vi "Emballage_BDD_lecture_Table_Correspondance_GVF_Index.vi"(10 "Column Names en entrée":string[](array[string]), 11 "Énum":enum16{"get", "set"}(ring)) -> (3 "Cluster_index_champs_correspondance":T1)   [LabVIEW 2020]
uses:
  Emballage_Index_correspondance.ctl
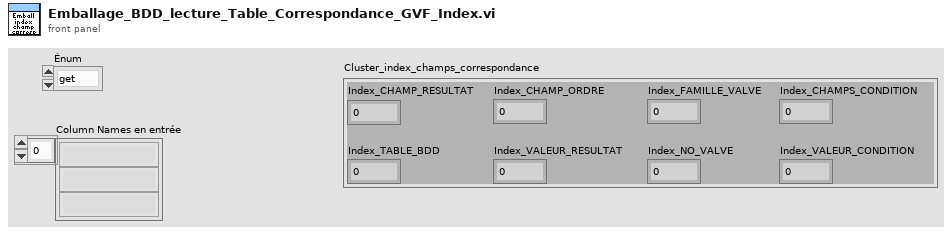
[diagram p1: front panel]
types:
  T1 = typedef "Emballage_Index_correspondance.ctl" = cluster{"Index_CHAMP_RESULTAT":i32, "Index_TABLE_BDD":i32, "Index_CHAMP_ORDRE":i32, "Index_VALEUR_RESULTAT":i32, "Index_FAMILLE_VALVE":i32, "Index_NO_VALVE":i32, "Index_CHAMPS_CONDITION":i32, "Index_VALEUR_CONDITION":i32}
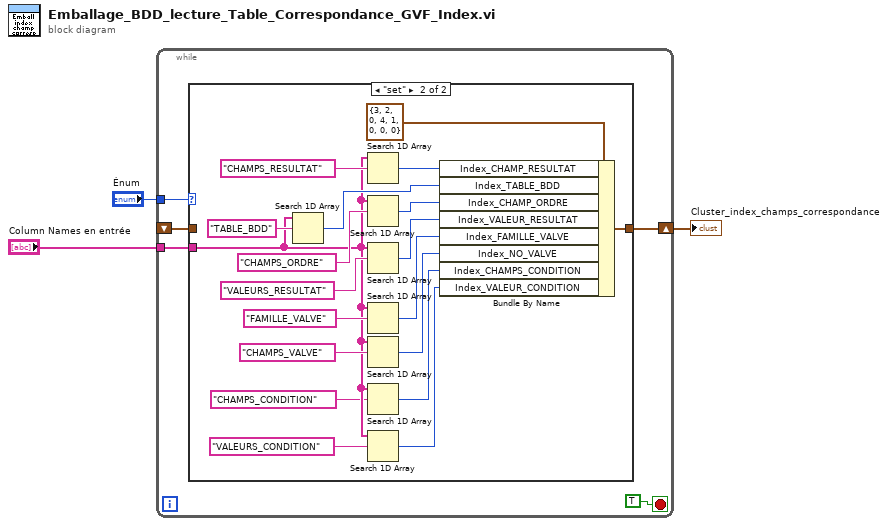
[diagram p0: block diagram]
diagram:
  n1 = while {
    tunnel: "Énum" -> [w7]
    shift-right: [w6] -> w2
    shift-left: _ -> [w5]
    tunnel: "Column Names en entrée" -> [w4]
    stop <- TRUE stop-if-true
    n2 = case shown="\"set\"" w7 {
      tunnel: [w9 w21] -> w6
      tunnel: w5 -> [w9 _]
      tunnel: w4 -> [_ w14]
      frame "get", Default {
      }
      frame "set" {
        n3 = Search 1D Array(1D array=w14, element="TABLE_BDD" ("élément")) -> (index of element=w17:i32)  [unwired: 1 in]
        n4 = Search 1D Array(1D array=w14, element="CHAMPS_RESULTAT" ("élément")) -> (index of element=w16:i32)  [unwired: 1 in]
        n5 = Search 1D Array(1D array=w14, element="CHAMPS_ORDRE" ("élément")) -> (index of element=w15:i32)  [unwired: 1 in]
        n6 = Search 1D Array(1D array=w14, element="VALEURS_RESULTAT" ("élément")) -> (index of element=w18:i32)  [unwired: 1 in]
        n7 = Search 1D Array(1D array=w14, element="FAMILLE_VALVE" ("élément")) -> (index of element=w19:i32)  [unwired: 1 in]
        n8 = Search 1D Array(1D array=w14, element="CHAMPS_VALVE" ("élément")) -> (index of element=w20:i32)  [unwired: 1 in]
        n9 = Search 1D Array(1D array=w14, element="CHAMPS_CONDITION" ("élément")) -> (index of element=w11:i32)  [unwired: 1 in]
        n10 = Search 1D Array(1D array=w14, element="VALEURS_CONDITION" ("élément")) -> (index of element=w10:i32)  [unwired: 1 in]
        n11 = Bundle By Name(cluster=T1 {"Index_CHAMP_RESULTAT"=3, "Index_TABLE_BDD"=2, "Index_CHAMP_ORDRE"=0, "Index_VALEUR_RESULTAT"=4, "Index_FAMILLE_VALVE"=1, "Index_NO_VALVE"=0, "Index_CHAMPS_CONDITION"=0, "Index_VALEUR_CONDITION"=0} ("Cluster_index_champs_correspondance"), "Index_CHAMP_RESULTAT"=w16, "Index_TABLE_BDD"=w17, "Index_CHAMP_ORDRE"=w15, "Index_VALEUR_RESULTAT"=w18, "Index_FAMILLE_VALVE"=w19, "Index_NO_VALVE"=w20, "Index_CHAMPS_CONDITION"=w11, "Index_VALEUR_CONDITION"=w10) -> (w21:T1)
      }
    }
  }
  "Cluster_index_champs_correspondance" <- w2
